vi "SplitStringIntoArrayOfStrings.vi"(11 "String":string) -> (3 "Characters":string[](array[string]))   [LabVIEW 2013, in "BarCodes.lvlib"]
doc: "Splits a VI in to an array of characters."
uses:
  BarCodes.lvlib
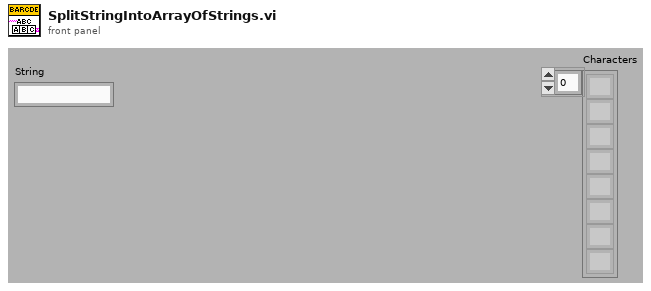
[diagram p1: front panel]
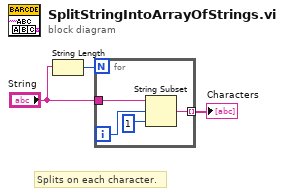
[diagram p0: block diagram]
diagram:
  # "Splits on each character."
  n1 = String Length(string="String") -> (length=w3:i32)
  n2 = for {
    N: w3 -> [_]
    tunnel: "String" -> [w7]
    tunnel: [w5] -> w1 mode=indexing
    i -> [w4]
    n3 = String Subset(string=w7, offset (0)=w4, length (rest)=1 ("length (rest)")) -> (substring=w5:string)
  }
  "Characters" <- w1
